vi "HandleError.vi"(0 "reference in":refnum<class "MB_MODULE.lvclass">, 11 "error in (no error)":errorcluster) -> (4 "reference out":refnum<class "MB_MODULE.lvclass">, 15 "error out":errorcluster)   [LabVIEW 2019, in "MB_MODULE.lvclass"]
uses:
  MB_MODULE.lvclass
  MB_MODULE.lvclass/MB_MODULE.ctl
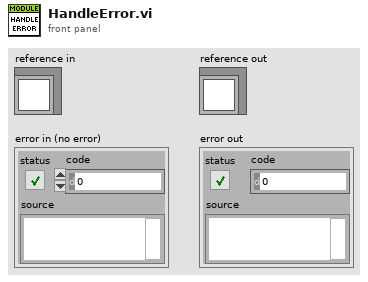
[diagram p1: front panel]
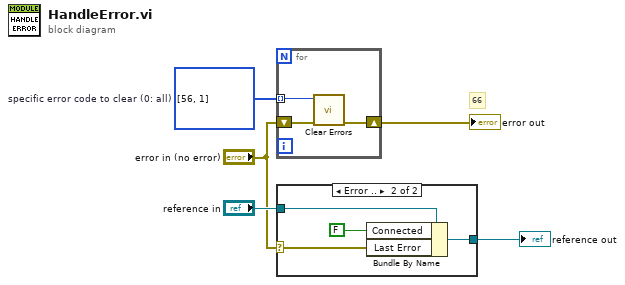
[diagram p0: block diagram]
diagram:
  w3 = i32[] [56, 1]  # specific error code to clear (0: all)
  # "66"
  n1 = for {
    shift-right: [w6] -> w2
    shift-left: "error in (no error)" -> [w8]
    tunnel: w3 -> [w7] mode=indexing
    n2 = call <vilib>:"Clear Errors.vi"("error in (no error)"=w8, "specific error code to clear (0: all)"=w7) -> ("error out"=w6:errorcluster)  [unwired: 4 in, 1 out]
  }
  "error out" <- w2
  n3 = case shown="Error .." "error in (no error)" {
    selector: "error in (no error)" -> [_ w10]
    tunnel: [w9 w13] -> w5
    tunnel: "reference in" -> [w9 w12]
    frame No Error {
    }
    frame Error {
      n4 = Bundle By Name(cluster=w12, "Connected"=FALSE, "Last Error"=w10) -> (w13:refnum<class "MB_MODULE.lvclass">)
    }
  }
  "reference out" <- w5
